vi "NATS Server Remove Windows.vi"() -> (0 "error out":errorcluster)   [LabVIEW 2024, in "NATS Infrastructure.lvlib"]
doc: "Starts NATS server on Windows machines."
uses:
  NATS Infrastructure.lvlib
panel:
  out "Return Code":i32
  out "Error":string
  out "Output":string
  in  "Install Directory":path=path "C:/nats"
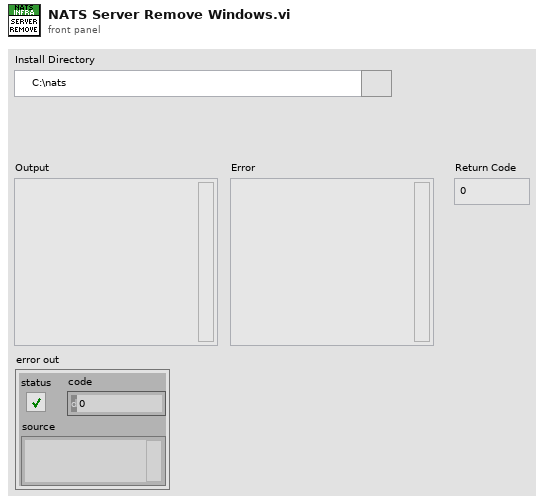
[diagram p1: front panel]
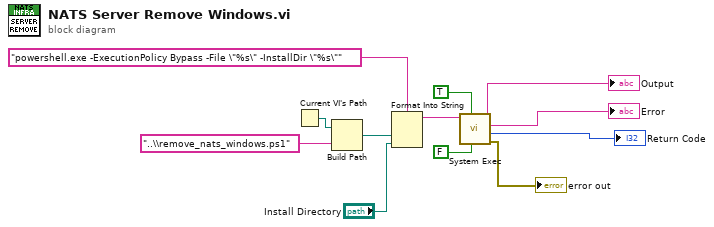
[diagram p0: block diagram]
diagram:
  n1 = Current VI's Path() -> (path=w7:path)
  n2 = Build Path(base path=w7, name or relative path="..\\remove_nats_windows.ps1") -> (appended path=w6:path)
  n3 = Format Into String(format string="powershell.exe -ExecutionPolicy Bypass -File \"%s\" -InstallDir \"%s\"", w6, "Install Directory") -> (resulting string=w5:string)  [unwired: 2 in, 1 out]
  n4 = call <vilib>:"System Exec.vi"("run minimized? (F)"=FALSE, "wait until completion? (T)"=TRUE, "command line"=w5) -> ("error out"=→"error out":errorcluster, "return code"=→"Return Code":i32, "standard error"=→"Error":string, "standard output"=→"Output":string)  [unwired: 5 in]
